vi "Okres.vi"(8 "error in (no error)":errorcluster, 9 "Offset":dbl, 10 "Uref":dbl, 11 "fclk-zad":dbl) -> (0 "error out":errorcluster, 3 "T1+T2":dbl)   [LabVIEW 2021]
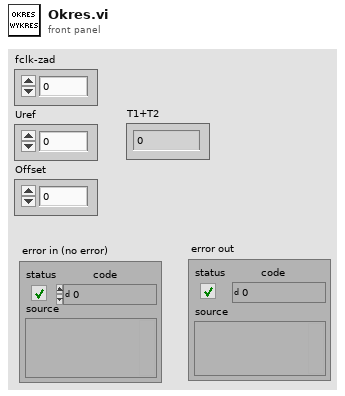
[diagram p1: front panel]
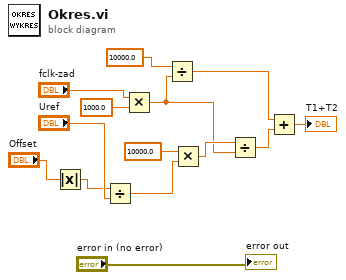
[diagram p0: block diagram]
diagram:
  n1 = Absolute Value(x="Offset") -> (abs(x)=w1:dbl)
  n2 = Divide(x=w1, y="Uref") -> (x/y=w10:dbl)
  n3 = Multiply(x="fclk-zad", y=1000.0) -> (x*y=w3:dbl)
  n4 = Divide(x=10000.0, y=w3) -> (x/y=w6:dbl)
  n5 = Multiply(x=10000.0, y=w10) -> (x*y=w9:dbl)
  n6 = Divide(x=w9, y=w3) -> (x/y=w7:dbl)
  n7 = Add(x=w6, y=w7) -> (x+y=→"T1+T2":dbl)
  "error out" <- "error in (no error)"
